vi "get configuration.vi"(8 "error in (no error)":errorcluster, 11 "shared memory editor node in":refnum<class "module editor node.lvclass">) -> (0 "error out":errorcluster, 2 "shm configuration out":refnum<class "Shared Memory configuration.lvclass">, 3 "shared memory editor node out":refnum<class "module editor node.lvclass">)   [LabVIEW 2014, in "Shared Memory editor node.lvclass"]
uses:
  Shared Memory editor node.lvclass
  <vilib>/NI/DCAF/Tag Editor Core/Configuration Editor/Classes/Module editor node/module editor node.lvclass
  module/configuration/Shared Memory configuration.lvclass
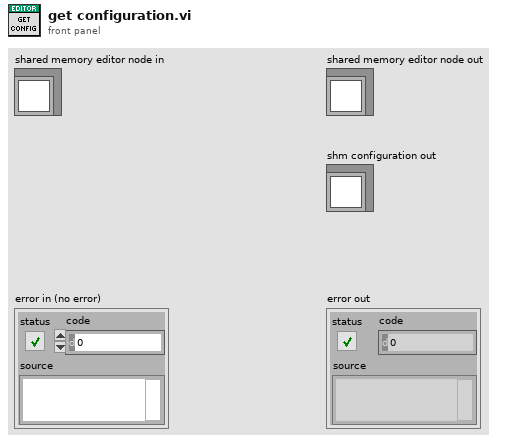
[diagram p1: front panel]
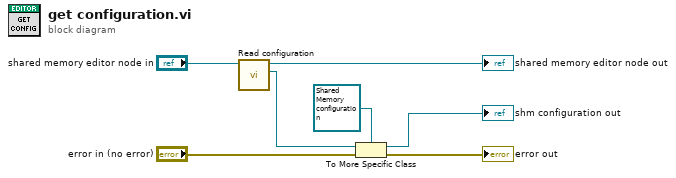
[diagram p0: block diagram]
diagram:
  n1 = call-dynamic "Read configuration.vi"("NISE_CEF_serializable node in"="shared memory editor node in") -> ("configuration"=w6:refnum<class "NISE_CEF_serializable configuration.lvclass">, "NISE_CEF_serializable node out"=→"shared memory editor node out":refnum<class "module editor node.lvclass">)  [unwired: 8 in, 1 out]
  n2 = To More Specific Class(target class=refnum<class "Shared Memory configuration.lvclass"> refnum ("shared memory configuration"), reference=w6, error in="error in (no error)") -> (specific class reference=→"shm configuration out":refnum<class "Shared Memory configuration.lvclass">, error out=→"error out":errorcluster)
